vi "Inst.RP100.setState.vi"(8 "error in (no error)":errorcluster, 10 "data in":variant, 11 "Inst.RP100 in":refnum<class "Inst.RP100.lvclass">) -> (0 "error out":errorcluster, 3 "Inst.RP100 out":refnum<class "Inst.RP100.lvclass">)   [LabVIEW 2019, in "Inst.RP100.lvclass"]
uses:
  Inst.RP100.lvclass
  Typedefs/Output Channel--Enum.ctl
  Typedefs/setOutput--Cluster.ctl
  Typedefs/Output State--Enum.ctl
  Inst.RP100.lvclass/Inst.RP100.ctl
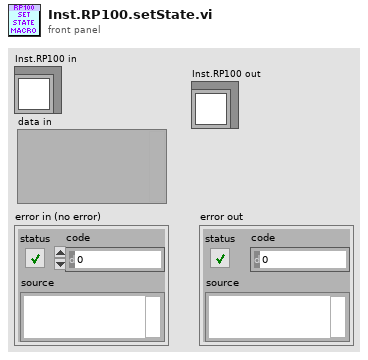
[diagram p1: front panel]
types:
  T1 = typedef "Inst.RP100.lvclass/setOutput--Cluster.ctl" = cluster{"State":T2}
  T2 = typedef "Inst.RP100.lvclass/Output State--Enum.ctl" = enum16{"Shorted", "Enabled"}
  T3 = typedef "Inst.RP100.lvclass/Output Channel--Enum.ctl" = enum16{"Output 1", "Output 2"}
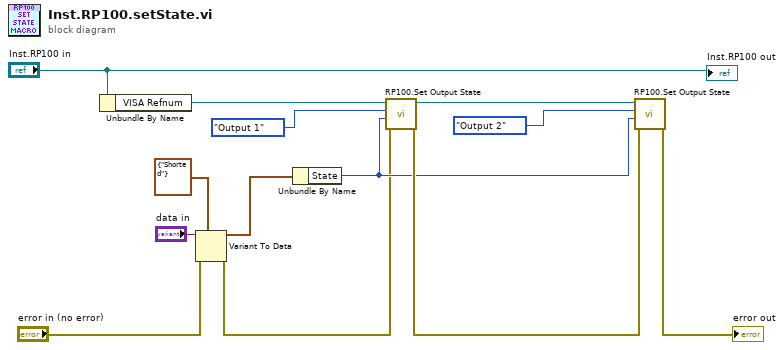
[diagram p0: block diagram]
diagram:
  n1 = Unbundle By Name("Inst.RP100 in") -> ("VISA Refnum"=w3:refnum<visa-resource-name>)
  n2 = Variant To Data(error in="error in (no error)", type=T1 {"State"=enum."Shorted"} ("Data out"), Variant="data in") -> (data=w5:T1, error out=w4:errorcluster)
  n3 = Unbundle By Name(w5) -> ("State"=w8:T2)
  n4 = call "RP100.Set Output State.vi"("error in (no error)"=w4, "Output State"=w8, "Output Channel"=Output_Channel--Enum."Output 1", "VISA resource name"=w3) -> ("error out"=w12:errorcluster, "VISA Refnum out"=w11:refnum<visa-resource-name>)  [unwired: 5 in, 1 out]
  n5 = call "RP100.Set Output State.vi"("error in (no error)"=w12, "Output State"=w8, "Output Channel"=Output_Channel--Enum."Output 2", "VISA resource name"=w11) -> ("error out"=→"error out":errorcluster)  [unwired: 5 in, 2 out]
  "Inst.RP100 out" <- "Inst.RP100 in"
